vi "XY Sub VI.vi"(6 "stop":bool, 7 "Movement\nComplete?":bool, 8 "error in (no error)":errorcluster, 9 "Y Axis Setpoint":T6, 10 "X Axis Setpoint":T4, 11 "Coordinates Input":T5={"X-axis (mm)"=0.0, "Y-axis (mm)"=0.0, "Y dist  target \nthreshold (mm)"=1.0, "X dist target\nthreshold (mm)"=0.0} {"X dist target\nthreshold (mm)" min=0.0; "Y dist  target \nthreshold (mm)" min=0.0}) -> (0 "error out":errorcluster, 1 "Y Path Display":T7, 2 "Y Axis":T8(graph), 3 "X Axis":T8(graph), 4 "Completed?":bool, 5 "Data Array":dbl[][](array[numeric]))   [LabVIEW 2017]
uses:
  Coords Input Cluster.ctl
  Encoder Cluster.ctl
  <vilib>/myRIO/Common/Instrument Driver Framework/myRIO v1.0/Encoder/typedefs/Encoder Count Direction Enum.ctl
  Motor Status Enum.ctl
panel:
  out "X Motor State":T1
  out "Y Motor State":T1
  out "Encoder Output":T2
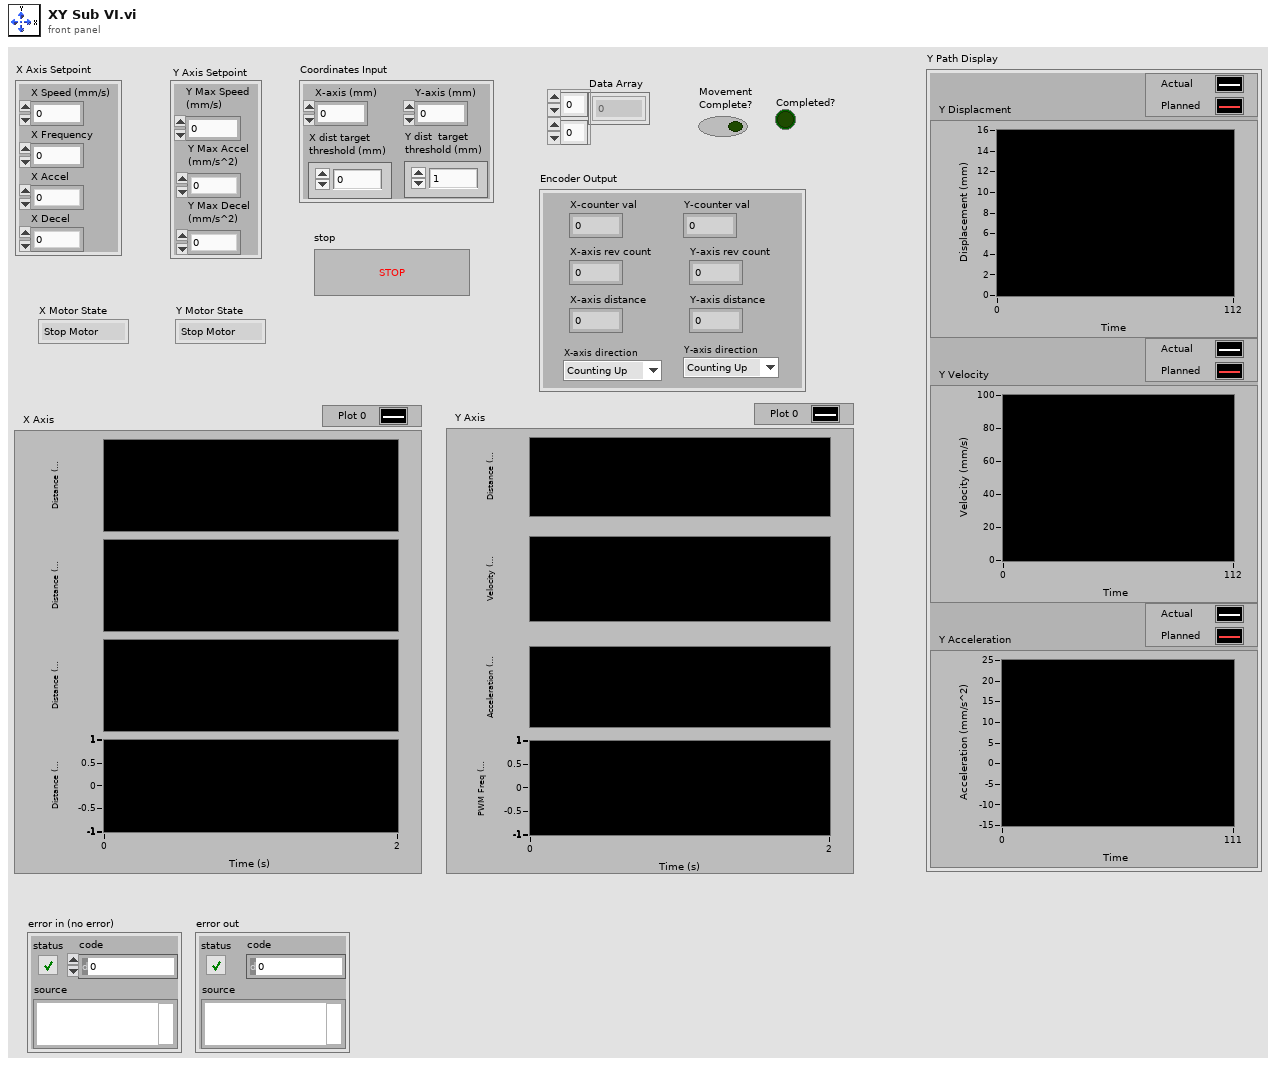
[diagram p1: front panel]
types:
  T1 = typedef "Motor Status Enum.ctl" = enum16{"Stop Motor", "Read Inputs", "Steady Speed", "Accelerate", "Decelerate"}
  T2 = typedef "Encoder Cluster.ctl" = cluster{"Y-axis rev count":dbl, "Y-axis distance":dbl, "X-axis rev count":dbl, "X-axis distance":dbl, "Y-axis direction":T3, "X-axis direction":T3, "X-counter val":i32, "Y-counter val":i32}
  T3 = typedef "Encoder Count Direction Enum.ctl" = enum16{"Counting Up", "Counting Down"}
  T4 = cluster{"X Frequency":dbl, "X Accel":dbl, "X Decel":dbl, "X Speed (mm/s)":dbl}
  T5 = typedef "Coords Input Cluster.ctl" = cluster{"X-axis (mm)":dbl, "Y-axis (mm)":dbl, "Y dist  target \nthreshold (mm)":dbl, "X dist target\nthreshold (mm)":dbl}
  T6 = cluster{"Y Max Speed \n(mm/s)":dbl, "Y Max Accel\n(mm/s^2)":dbl, "Y Max Decel \n(mm/s^2)":dbl}
  T7 = cluster{"Y Velocity":dbl[][], "Y Displacment":dbl[][], "Y Acceleration":dbl[][]}
  T8 = cluster{"X-axis distance":dbl, dbl, dbl, "X Frequency":dbl}
  T9 = cluster{"X Frequency":dbl, "X FWD/RVS":bool, "X Accel":dbl, "X Decel":dbl, "X Duty Cycle %":dbl}
  T10 = cluster{"Y Frequency":dbl, "Y FWD/RVS":bool, "Y Accel":dbl, "Y Decel":dbl}
  T11 = cluster{"Target Coords (mm)":dbl, "Current Coords (mm)":dbl, "Max Speed (mm/s)":dbl, "Max Accel (mm/s^2)":dbl, "Max Decel (mm/s^2)":dbl}
  T12 = cluster{" Distance target (mm)":dbl, "Max Accel (mm/s^2)":dbl, "Max Decel (mm/s^2)":dbl, "Velocity Limit (mm/s) ":dbl, "Time step (s)":dbl}
  T13 = enum16{"800", "1600", "3200", "6400", "12800", "25600"}
  T14 = cluster{"Cruising Speed (mm/s)":dbl, "Crusing Time (s)":dbl, "Decel Time (s)":dbl, "Accel Time (s)":dbl, "Total Time (s)":dbl, "Accel Distance (mm)":dbl, "Decel Distance (mm)":dbl, "Crusing Distance (mm)":dbl}
  T15 = cluster{"X-axis distance":dbl, dbl, dbl, "X Duty Cycle %":dbl}
  T16 = cluster{"Y-axis distance":dbl, dbl, dbl, "Y Frequency":dbl}
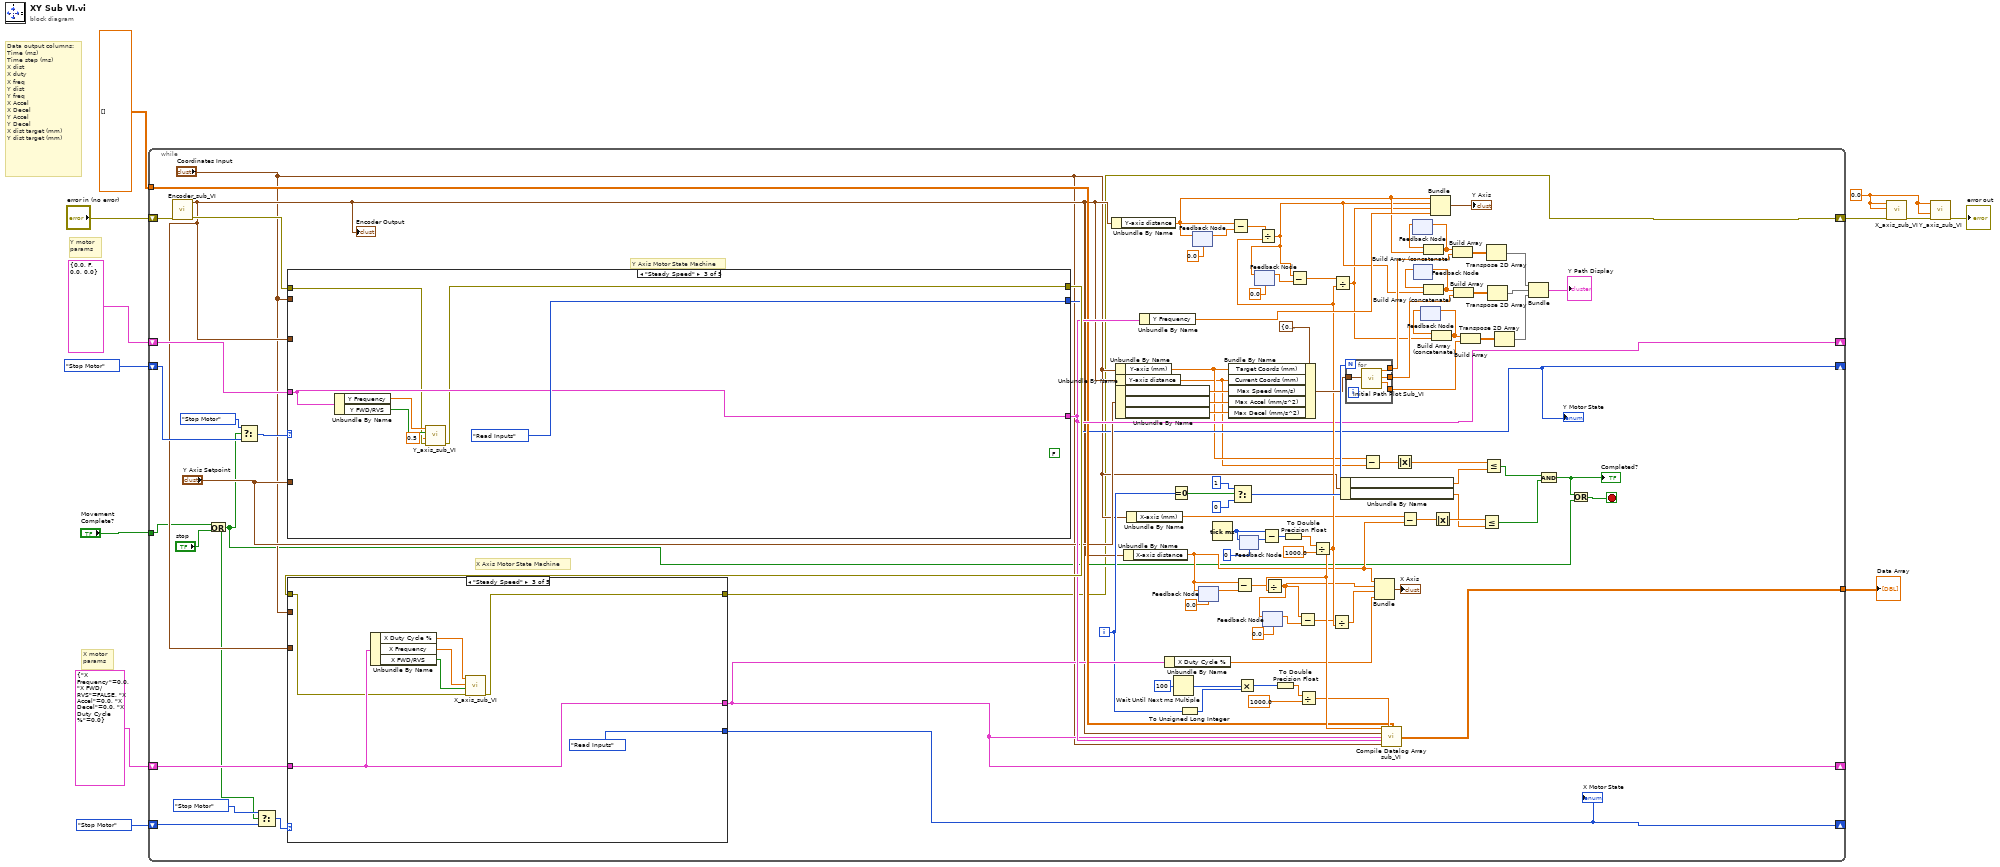
[diagram p0: block diagram]
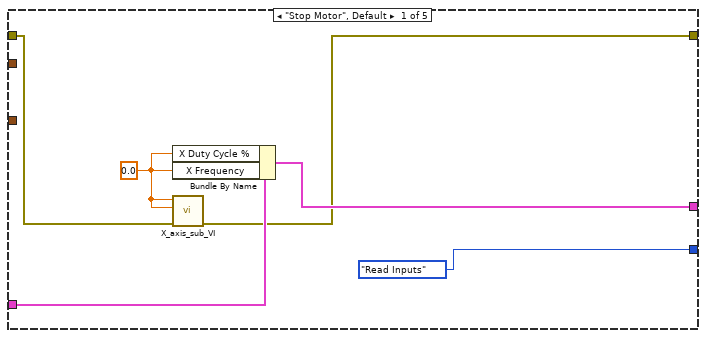
[diagram p2: hidden frame]
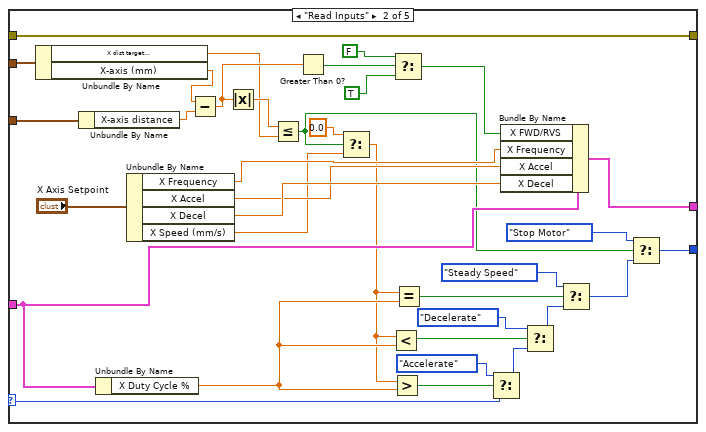
[diagram p3: hidden frame]
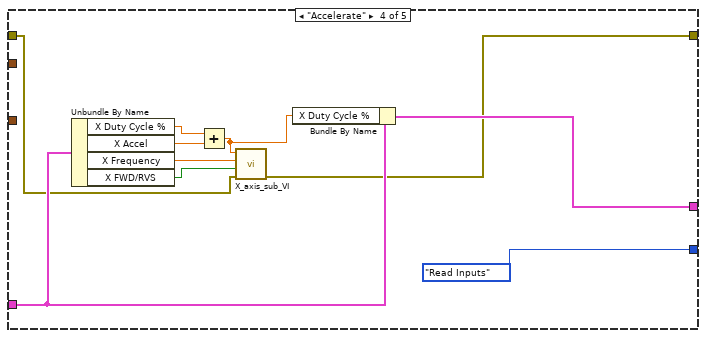
[diagram p4: hidden frame]
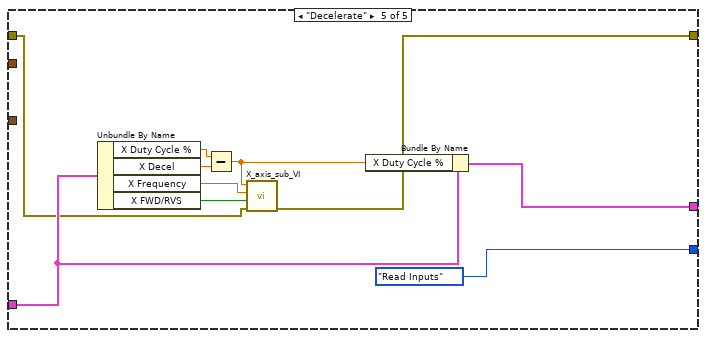
[diagram p5: hidden frame]
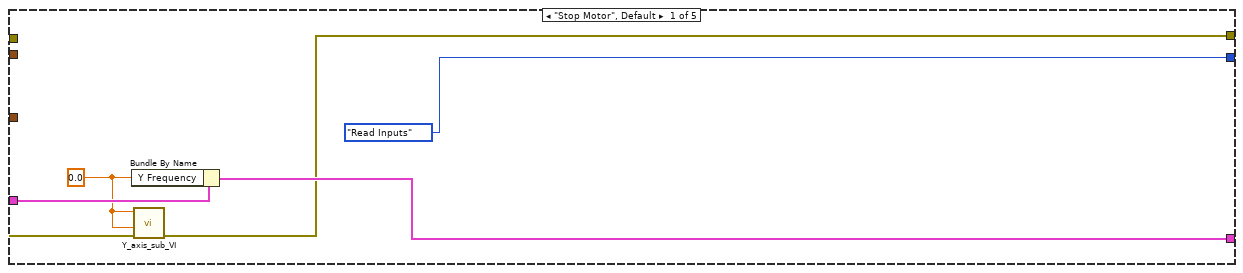
[diagram p6: hidden frame]
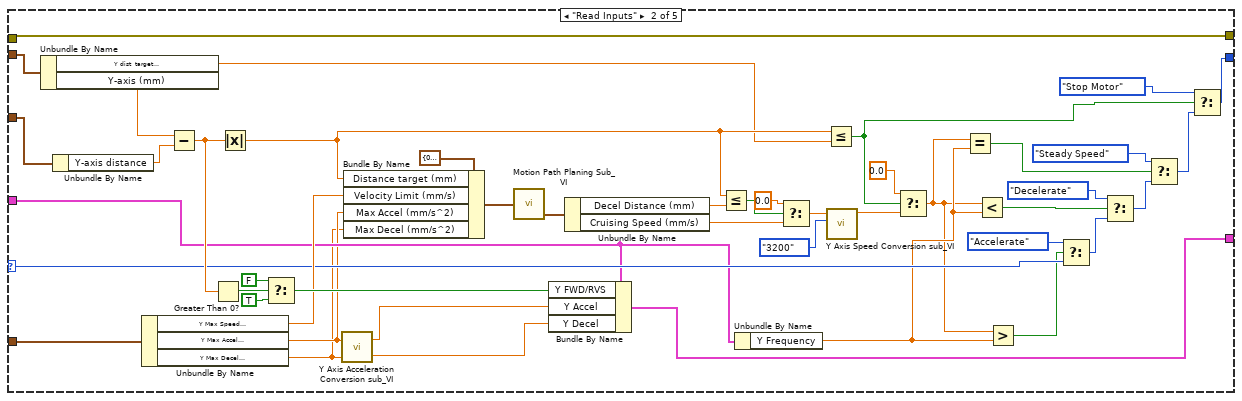
[diagram p7: hidden frame]
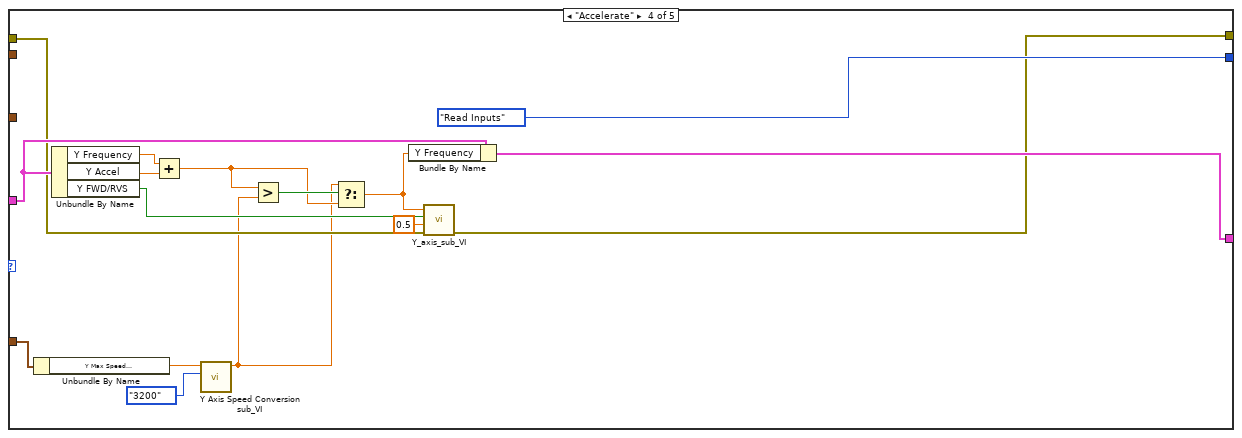
[diagram p8: hidden frame]
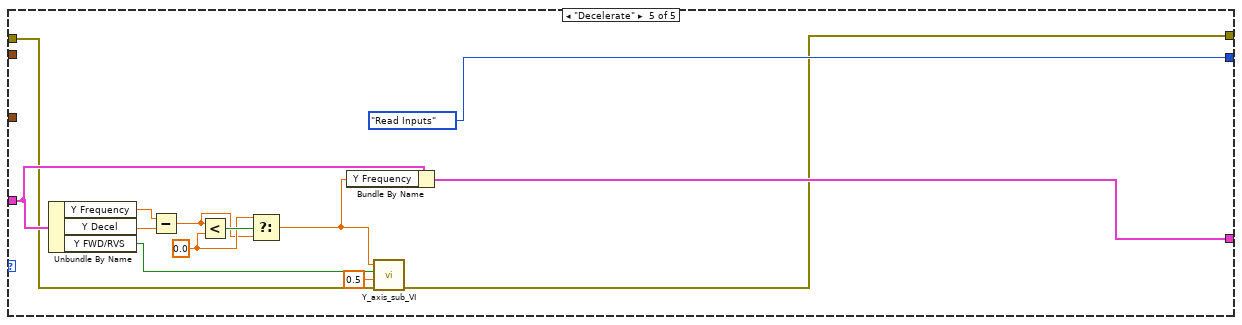
[diagram p9: hidden frame]
diagram:
  w4 = 0.0 ("Y Frequency")
  # "X motor \nparams"
  # "Y motor \nparams"
  # "Data output columns:\nTime (ms)\nTime step (ms)\nX dist\nX duty\nX freq\nY dist\nY freq\nX Accel\nX Decel\nY Accel\nY Decel\nX dist target (mm)\nY dist target (mm)"
  n1 = while {
    tunnel: [w52] -> w7
    shift-right: [w51] -> _
    shift-left: T10 {"Y Frequency"=0.0, "Y FWD/RVS"=FALSE, "Y Accel"=0.0, "Y Decel"=0.0} ("Y Axis Motor Params 2") -> [w44]
    shift-right: [w36] -> _
    shift-left: Motor_Status_Enum."Stop Motor" -> [w43]
    tunnel: dbl[][] [] -> [w42]
    shift-right: [w40] -> _
    shift-left: T9 {"X Frequency"=0.0, "X FWD/RVS"=FALSE, "X Accel"=0.0, "X Decel"=0.0, "X Duty Cycle %"=0.0} ("X Axis Motor Params 3") -> [w46]
    shift-right: [w37] -> _
    shift-left: Motor_Status_Enum."Stop Motor" -> [w45]
    shift-right: [w16] -> w3
    shift-left: "error in (no error)" -> [w38]
    tunnel: "Movement\nComplete?" -> [w21]
    i -> [w39]
    stop <- w18 stop-if-true
    w66 = u32 100 ("milliseconds to wait")
    # "X Axis Motor State Machine"
    # "Y Axis Motor State Machine"
    n2 = call "Encoder_sub_VI.vi"("error in (no error)"=w38) -> ("error out"=w88:errorcluster, "Encoder Output"=w32:T2)  [unwired: 9 in]
    "Encoder Output" <- w32
    n3 = Or(x=w21, y="stop") -> (x .or. y?=w19:bool)
    n4 = Select(t=Motor_Status_Enum."Stop Motor", s=w19, f=w43) -> (s? t:f=w55:T1)
    n5 = Select(t=Motor_Status_Enum."Stop Motor", s=w19, f=w45) -> (s? t:f=w58:T1)
    n6 = case shown="\"Steady Speed\"" w55 {
      selector: w55 -> [_ w205 _ _ _]
      tunnel: w44 -> [w188 w201 w238 w254 w266]
      tunnel: [Motor_Status_Enum."Read Inputs" w196 Motor_Status_Enum."Read Inputs" Motor_Status_Enum."Read Inputs" Motor_Status_Enum."Read Inputs"] -> w36
      tunnel: [w186 w194 w238 w253 w267] -> w51
      tunnel: w88 -> [w184 w207 w237 w251 w264]
      tunnel: [w185 w207 w236 w250 w265] -> w59
      tunnel: w32 -> [_ w209 _ _ _]
      tunnel: "Coordinates Input" -> [_ w208 _ _ _]
      tunnel: "Y Axis Setpoint" -> [_ w195 _ w249 _]
      frame "Stop Motor", Default {
        w183 = 0.0 ("Y Frequency")
        n7 = Bundle By Name(cluster=w188, "Y Frequency"=w183) -> (w186:T10)
        n8 = call "Y_axis_sub_VI.vi"("error in (no error)"=w184, "Duty Cycle"=w183, "Frequency"=w183) -> ("error out"=w185:errorcluster)  [unwired: 8 in]
      }
      frame "Read Inputs" {
        n9 = Unbundle By Name(w208) -> ("Y dist  target \nthreshold (mm)"=w190:dbl, "Y-axis (mm)"=w220:dbl)
        n10 = Unbundle By Name(w209) -> ("Y-axis distance"=w219:dbl)
        n11 = Unbundle By Name(w195) -> ("Y Max Speed \n(mm/s)"=w206:dbl, "Y Max Accel\n(mm/s^2)"=w193:dbl, "Y Max Decel \n(mm/s^2)"=w192:dbl)
        n12 = Subtract(x=w220, y=w219) -> (x-y=w216:dbl)
        n13 = Greater Than 0?(x=w216) -> (x > 0?=w224:bool)
        n14 = Absolute Value(x=w216) -> (abs(x)=w200:dbl)
        n15 = Select(t=FALSE, s=w224, f=TRUE) -> (s? t:f=w225:bool)
        n16 = call "Y Axis Acceleration Conversion sub_VI.vi"("Deceleration (mm/s^2)"=w192, "Acceleration (mm/s^2)"=w193) -> ("Freq decrease per 0.1ms (Hz)"=w210:dbl, "Freq increase per 0.1ms (Hz)"=w211:dbl)
        n17 = Bundle By Name(cluster=T12 {" Distance target (mm)"=0.0, "Max Accel (mm/s^2)"=0.0, "Max Decel (mm/s^2)"=0.0, "Velocity Limit (mm/s) "=0.0, "Time step (s)"=0.0} ("Motion Planning Inputs"), "Distance target (mm)"=w200, "Velocity Limit (mm/s)"=w206, "Max Accel (mm/s^2)"=w193, "Max Decel (mm/s^2)"=w192) -> (w218:T12)
        n18 = call "Motion Path Planing Sub_VI.vi"("Motion Planning Inputs"=w218) -> ("Motion Planning Outputs"=w191:T14)  [unwired: 4 in, 2 out]
        n19 = Bundle By Name(cluster=w201, "Y FWD/RVS"=w225, "Y Accel"=w211, "Y Decel"=w210) -> (w194:T10)
        n20 = Unbundle By Name(w191) -> ("Decel Distance (mm)"=w215:dbl, "Cruising Speed (mm/s)"=w203:dbl)
        n21 = Less Or Equal?(x=w200, y=w215) -> (x <= y?=w214:bool)
        n22 = Unbundle By Name(w201) -> ("Y Frequency"=w202:dbl)
        n23 = Select(t=0.0, s=w214, f=w203) -> (s? t:f=w212:dbl)
        n24 = Less Or Equal?(x=w200, y=w190) -> (x <= y?=w189:bool)
        n25 = call "Y Axis Speed Conversion sub_VI.vi"("Microsteps per Rev"=T13."3200", "Setpoint\nSpeed (mm/s)"=w212) -> ("PWM Frequency"=w222:dbl)  [unwired: 9 in]
        n26 = Select(t=0.0, s=w189, f=w222) -> (s? t:f=w199:dbl)
        n27 = Equal?(x=w199, y=w202) -> (x = y?=w232:bool)
        n28 = Less?(x=w199, y=w202) -> (x < y?=w229:bool)
        n29 = Greater?(x=w199, y=w202) -> (0:w204:bool)
        n30 = Select(t=Motor_Status_Enum."Accelerate", s=w204, f=w205) -> (s? t:f=w231:T1)
        n31 = Select(t=Motor_Status_Enum."Decelerate", s=w229, f=w231) -> (s? t:f=w233:T1)
        n32 = Select(t=Motor_Status_Enum."Steady Speed", s=w232, f=w233) -> (s? t:f=w197:T1)
        n33 = Select(t=Motor_Status_Enum."Stop Motor", s=w189, f=w197) -> (s? t:f=w196:T1)
      }
      frame "Steady Speed" {
        (unwired) FALSE
        n34 = Unbundle By Name(w238) -> ("Y Frequency"=w240:dbl, "Y FWD/RVS"=w241:bool)
        n35 = call "Y_axis_sub_VI.vi"("error in (no error)"=w237, "Duty Cycle"=0.5, "FWD/RVS"=w241, "Frequency"=w240) -> ("error out"=w236:errorcluster)  [unwired: 7 in]
      }
      frame "Accelerate" {
        n36 = Unbundle By Name(w249) -> ("Y Max Speed \n(mm/s)"=w244:dbl)
        n37 = Unbundle By Name(w254) -> ("Y Frequency"=w256:dbl, "Y Accel"=w257:dbl, "Y FWD/RVS"=w252:bool)
        n38 = Add(x=w256, y=w257) -> (x+y=w247:dbl)
        n39 = call "Y Axis Speed Conversion sub_VI.vi"("Microsteps per Rev"=T13."3200", "Setpoint\nSpeed (mm/s)"=w244) -> ("PWM Frequency"=w243:dbl)  [unwired: 9 in]
        n40 = Greater?(x=w247, y=w243) -> (0:w248:bool)
        n41 = Select(t=w243, s=w248, f=w247) -> (s? t:f=w246:dbl)
        n42 = Bundle By Name(cluster=w254, "Y Frequency"=w246) -> (w253:T10)
        n43 = call "Y_axis_sub_VI.vi"("error in (no error)"=w251, "Duty Cycle"=0.5, "FWD/RVS"=w252, "Frequency"=w246) -> ("error out"=w250:errorcluster)  [unwired: 7 in]
      }
      frame "Decelerate" {
        w261 = 0.0 ("y")
        n44 = Unbundle By Name(w266) -> ("Y Frequency"=w270:dbl, "Y Decel"=w269:dbl, "Y FWD/RVS"=w263:bool)
        n45 = Subtract(x=w270, y=w269) -> (x-y=w260:dbl)
        n46 = Less?(x=w260, y=w261) -> (x < y?=w262:bool)
        n47 = Select(t=w261, s=w262, f=w260) -> (s? t:f=w259:dbl)
        n48 = Bundle By Name(cluster=w266, "Y Frequency"=w259) -> (w267:T10)
        n49 = call "Y_axis_sub_VI.vi"("error in (no error)"=w264, "Duty Cycle"=0.5, "FWD/RVS"=w263, "Frequency"=w259) -> ("error out"=w265:errorcluster)  [unwired: 7 in]
      }
    }
    "Y Motor State" <- w36
    n50 = case shown="\"Steady Speed\"" w58 {
      selector: w58 -> [_ w143 _ _ _]
      tunnel: [Motor_Status_Enum."Read Inputs" w123 Motor_Status_Enum."Read Inputs" Motor_Status_Enum."Read Inputs" Motor_Status_Enum."Read Inputs"] -> w37
      tunnel: [w117 w142 w159 w167 w176] -> w40
      tunnel: w46 -> [w118 w141 w159 w166 w175]
      tunnel: w59 -> [w116 w140 w157 w165 w174]
      tunnel: [w115 w140 w156 w164 w173] -> w16
      tunnel: w32 -> [_ w139 _ _ _]
      tunnel: "Coordinates Input" -> [_ w138 _ _ _]
      frame "Stop Motor", Default {
        w120 = 0.0 ("Y Frequency")
        n51 = Bundle By Name(cluster=w118, "X Duty Cycle %"=w120, "X Frequency"=w120) -> (w117:T9)
        n52 = call "X_axis_sub_VI.vi"("error in (no error)"=w116, "Frequency"=w120, "Duty Cycle %"=w120) -> ("error out"=w115:errorcluster)  [unwired: 8 in]
      }
      frame "Read Inputs" {
        n53 = Unbundle By Name(w138) -> ("X dist target\nthreshold (mm)"=w126:dbl, "X-axis (mm)"=w130:dbl)
        n54 = Unbundle By Name(w139) -> ("X-axis distance"=w129:dbl)
        n55 = Unbundle By Name(w141) -> ("X Duty Cycle %"=w154:dbl)
        n56 = Unbundle By Name("X Axis Setpoint") -> ("X Frequency"=w146:dbl, "X Accel"=w144:dbl, "X Decel"=w145:dbl, "X Speed (mm/s)"=w134:dbl)
        n57 = Subtract(x=w130, y=w129) -> (x-y=w128:dbl)
        n58 = Absolute Value(x=w128) -> (abs(x)=w127:dbl)
        n59 = Less Or Equal?(x=w127, y=w126) -> (x <= y?=w122:bool)
        n60 = Greater Than 0?(x=w128) -> (x > 0?=w136:bool)
        n61 = Select(t=0.0, s=w122, f=w134) -> (s? t:f=w133:dbl)
        n62 = Less?(x=w133, y=w154) -> (x < y?=w149:bool)
        n63 = Greater?(x=w133, y=w154) -> (0:w147:bool)
        n64 = Select(t=FALSE, s=w136, f=TRUE) -> (s? t:f=w131:bool)
        n65 = Equal?(x=w133, y=w154) -> (x = y?=w153:bool)
        n66 = Select(t=Motor_Status_Enum."Accelerate", s=w147, f=w143) -> (s? t:f=w151:T1)
        n67 = Bundle By Name(cluster=w141, "X FWD/RVS"=w131, "X Frequency"=w146, "X Accel"=w144, "X Decel"=w145) -> (w142:T9)
        n68 = Select(t=Motor_Status_Enum."Decelerate", s=w149, f=w151) -> (s? t:f=w152:T1)
        n69 = Select(t=Motor_Status_Enum."Steady Speed", s=w153, f=w152) -> (s? t:f=w124:T1)
        n70 = Select(t=Motor_Status_Enum."Stop Motor", s=w122, f=w124) -> (s? t:f=w123:T1)
      }
      frame "Steady Speed" {
        n71 = Unbundle By Name(w159) -> ("X Duty Cycle %"=w161:dbl, "X Frequency"=w160:dbl, "X FWD/RVS"=w162:bool)
        n72 = call "X_axis_sub_VI.vi"("error in (no error)"=w157, "FWD/RVS"=w162, "Frequency"=w160, "Duty Cycle %"=w161) -> ("error out"=w156:errorcluster)  [unwired: 7 in]
      }
      frame "Accelerate" {
        n73 = Unbundle By Name(w166) -> ("X Duty Cycle %"=w169:dbl, "X Accel"=w170:dbl, "X Frequency"=w171:dbl, "X FWD/RVS"=w163:bool)
        n74 = Add(x=w169, y=w170) -> (x+y=w172:dbl)
        n75 = call "X_axis_sub_VI.vi"("error in (no error)"=w165, "FWD/RVS"=w163, "Frequency"=w171, "Duty Cycle %"=w172) -> ("error out"=w164:errorcluster)  [unwired: 7 in]
        n76 = Bundle By Name(cluster=w166, "X Duty Cycle %"=w172) -> (w167:T9)
      }
      frame "Decelerate" {
        n77 = Unbundle By Name(w175) -> ("X Duty Cycle %"=w178:dbl, "X Decel"=w179:dbl, "X Frequency"=w180:dbl, "X FWD/RVS"=w182:bool)
        n78 = Subtract(x=w178, y=w179) -> (x-y=w181:dbl)
        n79 = call "X_axis_sub_VI.vi"("error in (no error)"=w174, "FWD/RVS"=w182, "Frequency"=w180, "Duty Cycle %"=w181) -> ("error out"=w173:errorcluster)  [unwired: 7 in]
        n80 = Bundle By Name(cluster=w175, "X Duty Cycle %"=w181) -> (w176:T9)
      }
    }
    "X Motor State" <- w37
    n81 = Unbundle By Name(w32) -> ("Y-axis distance"=w15:dbl)
    n82 = Unbundle By Name("Coordinates Input") -> ("Y-axis (mm)"=w35:dbl)
    n83 = Unbundle By Name(w32) -> ("Y-axis distance"=w34:dbl)
    n84 = Unbundle By Name("Y Axis Setpoint") -> ("Y Max Speed \n(mm/s)"=w91:dbl, "Y Max Accel\n(mm/s^2)"=w92:dbl, "Y Max Decel \n(mm/s^2)"=w93:dbl)
    n85 = Unbundle By Name(w32) -> ("X-axis distance"=w33:dbl)
    n86 = Unbundle By Name("Coordinates Input") -> ("X-axis (mm)"=w30:dbl)
    n87 = Unbundle By Name(w51) -> ("Y Frequency"=w110:dbl)
    n88 = Unbundle By Name(w40) -> ("X Duty Cycle %"=w71:dbl)
    n89 = Equal To 0?(x=w39) -> (x = 0?=w94:bool)
    n90 = Wait Until Next ms Multiple(millisecond multiple=w66) -> ()  [unwired: 1 out]
    n91 = To Unsigned Long Integer(number=w39) -> (unsigned 32bit integer=w67:u32)
    n92 = feedback #1(0.0) -> (w73:dbl)
    n93 = feedback-in #1(w15) -> ()
    n94 = feedback #2(0.0) -> (w79:dbl)
    n95 = feedback-in #2(w33) -> ()
    n96 = Tick Count (ms)() -> (millisecond timer value=w64:u32)
    n97 = Bundle By Name(cluster=T11 {"Target Coords (mm)"=0.0, "Current Coords (mm)"=0.0, "Max Speed (mm/s)"=0.0, "Max Accel (mm/s^2)"=0.0, "Max Decel (mm/s^2)"=0.0} ("Motion Inputs"), "Target Coords (mm)"=w35, "Current Coords (mm)"=w34, "Max Speed (mm/s)"=w91, "Max Accel (mm/s^2)"=w92, "Max Decel (mm/s^2)"=w93) -> (w90:T11)
    n98 = Subtract(x=w15, y=w73) -> (x-y=w74:dbl)
    n99 = Select(t=1, s=w94, f=0) -> (s? t:f=w95:i32)
    n100 = Subtract(x=w33, y=w79) -> (x-y=w80:dbl)
    n101 = Multiply(x=w66, y=w67) -> (x*y=w68:u32)
    n102 = feedback #3(u32 0) -> (w65:u32)
    n103 = feedback-in #3(w64) -> ()
    n104 = feedback #4(0.0) -> (w76:dbl)
    n105 = Subtract(x=w64, y=w65) -> (x-y=w61:u32)
    n106 = feedback #5(0.0) -> (w82:dbl)
    n107 = To Double Precision Float(number=w68) -> (double precision float=w69:dbl)
    n108 = To Double Precision Float(number=w61) -> (double precision float=w63:dbl)
    n109 = Divide(x=w69, y=1000.0) -> (x/y=w70:dbl)
    n110 = Divide(x=w63, y=1000.0) -> (x/y=w86:dbl)
    n111 = Divide(x=w74, y=w86) -> (x/y=w14:dbl)
    n112 = feedback-in #4(w14) -> ()
    n113 = Divide(x=w80, y=w86) -> (x/y=w84:dbl)
    n114 = feedback-in #5(w84) -> ()
    n115 = Subtract(x=w14, y=w76) -> (x-y=w77:dbl)
    n116 = Subtract(x=w84, y=w82) -> (x-y=w83:dbl)
    n117 = Divide(x=w83, y=w86) -> (x/y=w85:dbl)
    n118 = Divide(x=w77, y=w86) -> (x/y=w13:dbl)
    n119 = Unbundle By Name("Coordinates Input") -> ("Y dist  target \nthreshold (mm)"=w27:dbl, "X dist target\nthreshold (mm)"=w22:dbl)
    n120 = for {
      N: w95 -> [_]
      tunnel: w90 -> [w114]
      tunnel: [w113] -> w100
      tunnel: [w112] -> w105
      tunnel: [w111] -> w109
      n121 = call "Initial Path Plot Sub_VI.vi"("Motion Inputs"=w114) -> ("Accel Array"=w111:dbl[], "Velocity Array"=w113:dbl[], "Displacement Array"=w112:dbl[])  [unwired: 3 in, 5 out]
    }
    n122 = Subtract(x=w35, y=w34) -> (x-y=w29:dbl)
    n123 = Bundle("X-axis distance"=w33, w84, w85, "X Duty Cycle %"=w71) -> (→"X Axis":T15)  [unwired: 1 in]
    n124 = call "Compile Datalog Array sub_VI.vi"("Loop Runtime (s)"=w86, "Total Runtime (s)"=w70, "Initialised Array"=w42, "Encoder Output"=w32, "X Axis Motor Params"=w40, "Y Axis Motor Params"=w51, "Coordinates Input"="Coordinates Input") -> ("Data Array"=w52:dbl[][])  [unwired: 8 in]
    n125 = Absolute Value(x=w29) -> (abs(x)=w28:dbl)
    n126 = Subtract(x=w30, y=w33) -> (x-y=w25:dbl)
    n127 = feedback #6() -> (w104:dbl[])  [unwired: 1 in]
    n128 = feedback #7() -> (w98:dbl[])  [unwired: 1 in]
    n129 = feedback #8() -> (w108:dbl[])  [unwired: 1 in]
    n130 = Build Array (concatenate)(w104, w15) -> (w103:dbl[])
    n131 = feedback-in #6(w103) -> ()
    n132 = Build Array (concatenate)(w98, w14) -> (w99:dbl[])
    n133 = feedback-in #7(w99) -> ()
    n134 = Bundle("Y-axis distance"=w15, w14, w13, "Y Frequency"=w110) -> (→"Y Axis":T16)  [unwired: 1 in]
    n135 = Build Array (concatenate)(w108, w13) -> (w107:dbl[])
    n136 = feedback-in #8(w107) -> ()
    n137 = Absolute Value(x=w25) -> (abs(x)=w24:dbl)
    n138 = Build Array(w103, w105) -> (w102:dbl[][])
    n139 = Build Array(w99, w100) -> (w101:dbl[][])
    n140 = Build Array(w107, w109) -> (w106:dbl[][])
    n141 = Less Or Equal?(x=w24, y=w22) -> (x <= y?=w23:bool)
    n142 = Less Or Equal?(x=w28, y=w27) -> (x <= y?=w26:bool)
    n143 = Transpose 2D Array(2D array=w102) -> (transposed array=w49:dbl[][])
    n144 = Transpose 2D Array(2D array=w101) -> (transposed array=w48:dbl[][])
    n145 = Transpose 2D Array(2D array=w106) -> (transposed array=w47:dbl[][])
    n146 = Bundle(w49, w48, w47) -> (→"Y Path Display":cluster{dbl[][], dbl[][], dbl[][]})  [unwired: 1 in]
    n147 = And(x=w26, y=w23) -> (x .and. y?=w17:bool)
    "Completed?" <- w17
    n148 = Or(x=w17, y=w19) -> (x .or. y?=w18:bool)
  }
  "Data Array" <- w7
  n149 = call "X_axis_sub_VI.vi"("error in (no error)"=w3, "Frequency"=w4, "Duty Cycle %"=w4) -> ("error out"=w2:errorcluster)  [unwired: 8 in]
  n150 = call "Y_axis_sub_VI.vi"("error in (no error)"=w2, "Duty Cycle"=w4, "Frequency"=w4) -> ("error out"=→"error out":errorcluster)  [unwired: 8 in]
